vi "ReadJSON.vi"(11 "Key":string) -> (2 "Val_str":string, 3 "Val_num":dbl)   [LabVIEW 2017]
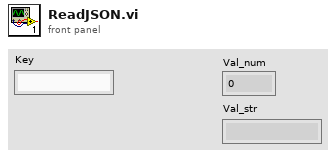
[diagram p1: front panel]
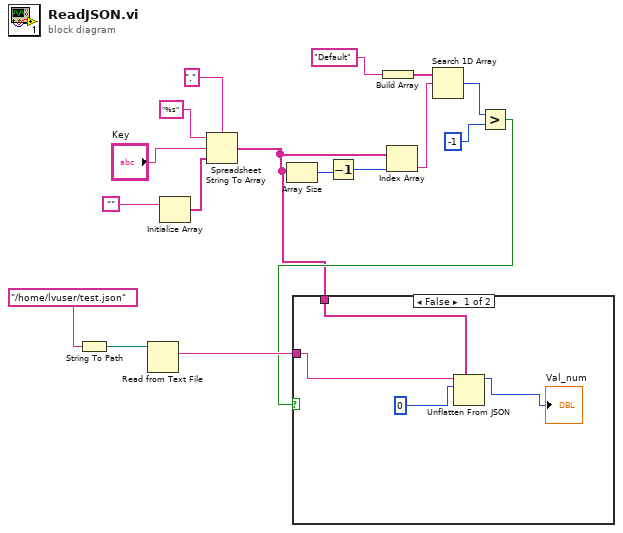
[diagram p0: block diagram]
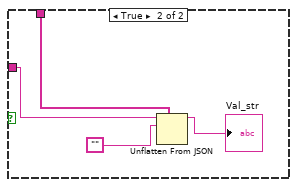
[diagram p2: hidden frame]
diagram:
  n1 = String To Path(string="/home/lvuser/test.json") -> (path=w16:path)
  n2 = Read from Text File(file (use dialog)=w16) -> (text=w17:string)  [unwired: 3 in, 3 out]
  n3 = Initialize Array("") -> (w12:string[])  [unwired: 1 in]
  n4 = Spreadsheet String To Array(delimiter (Tab)=".", format string="%s", spreadsheet string="Key", array type (2D Dbl)=w12) -> (array=w2:string[])
  n5 = Array Size(array=w2) -> (size(s)=w10:i32)
  n6 = Decrement(x=w10) -> (x-1=w7:i32)
  n7 = Build Array("Default") -> (w8:string[])
  n8 = Index Array(array=w2, index=w7) -> (element=w6:string)
  n9 = Search 1D Array(1D array=w8, element=w6) -> (index of element=w4:i32)  [unwired: 1 in]
  n10 = Greater?(x=w4, y=-1) -> (0:w3:bool)
  n11 = case shown="False" w3 {
    tunnel: w17 -> [w21 w23]
    tunnel: w2 -> [w18 w22]
    frame False {
      n12 = Unflatten From JSON(path=w18, JSON string=w21, type and defaults=0) -> (value=→"Val_num":i32)  [unwired: 4 in, 1 out]
    }
    frame True {
      n13 = Unflatten From JSON(path=w22, JSON string=w23, type and defaults="") -> (value=→"Val_str":string)  [unwired: 4 in, 1 out]
    }
  }
